vi "test subpanels.vi"() -> ()   [LabVIEW 2010]
uses:
  Stamp Controls.ctl
  switches.ctl
panel:
  out "Current Control settings":T1 {"Pump speed" format="%.2f"}
  in  "stop":bool
  in  "vi path":path
  # "rpm"
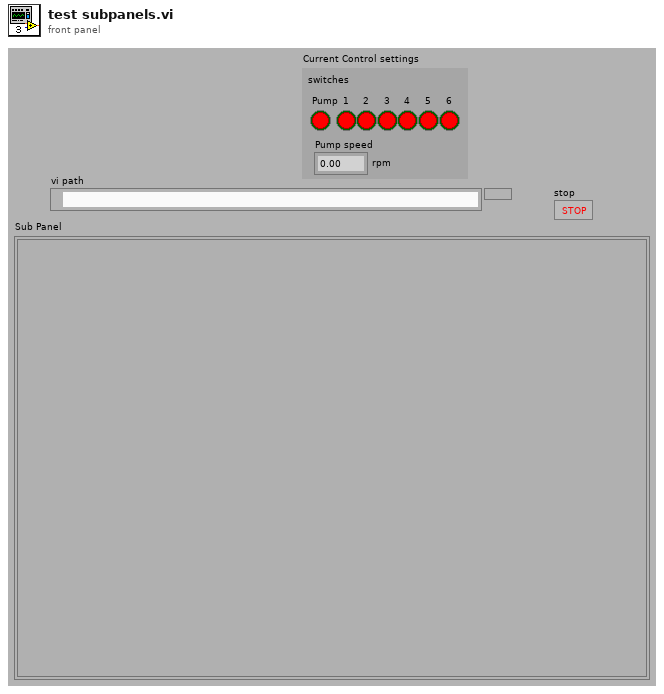
[diagram p1: front panel]
types:
  T1 = typedef "Stamp Controls.ctl" = cluster{"Pump speed":dbl, "switches":T2}
  T2 = typedef "switches.ctl" = cluster{"Pump":bool, "1":bool, "2":bool, "3":bool, "4":bool, "5":bool, "6":bool}
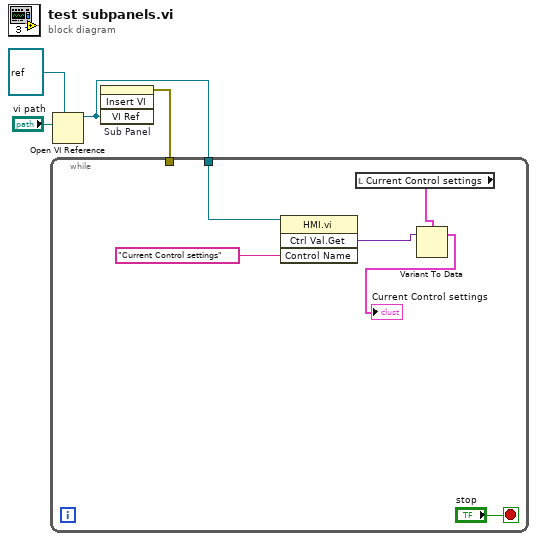
[diagram p0: block diagram]
diagram:
  n1 = Open VI Reference(type specifier VI Refnum (for type only)=refnum<vi> refnum, vi path="vi path") -> (vi reference=w1:refnum<vi>)  [unwired: 4 in, 1 out]
  n2 = invoke on="Sub Panel" class="SubPanel" method="Insert VI"("VI Ref"=w1) -> (error out=w2:errorcluster)  [unwired: 3 in, 3 out]
  n3 = while {
    tunnel: w2 -> [_]
    tunnel: w1 -> [w8]
    stop <- "stop" stop-if-true
    n4 = invoke class="HMI.vi" method="Ctrl Val.Get"(reference=w8, "Control Name"="Current Control settings") -> ("Get Control Value Variant"=w7:variant)  [unwired: 2 in, 3 out]
    n5 = local read "Current Control settings"() -> (w6:T1)
    n6 = Variant To Data(Variant=w7, type=w6) -> (data=→"Current Control settings":T1)  [unwired: 1 in, 1 out]
  }
